vi "Teleop.vi"(10 "Match Info":T1={"Autonomous Elapsed Seconds"=0.0, "TeleOp Elapsed Seconds"=0.0, "Disabled Elapsed Seconds"=0.0, "Visited Autonomous"=FALSE, "Visited TeleOp"=FALSE, "Visited Disabled"=FALSE, "Autonomous Settings"={"Autonomous Style"=enum."Independent", "VI Refnum"=refnum}}, 11 "Call Context":T2) -> ()   [LabVIEW 2019]
doc: "This VI is called for each TeleOp packet received from the DS where the robot is not disabled. It is often used to read from the joysticks and update I/O or to update setpoints for timed control loops. It should complete and return within 20 milliseconds or it may miss DS packets."
uses:
  ArgosLib/ArgosLib.lvlib
  InfiniteRechargeSrc/Global_Var-RefNum/JoystickControls.vi
  InfiniteRechargeSrc/TypeDefs/JoystickControl.ctl
  <vilib>/Rock Robotics/WPI/DriverStation/WPI_DriverStationMatch Info.ctl
  <vilib>/Rock Robotics/WPI/DriverStation/WPI_DriverStationDerivedRobotMode.ctl
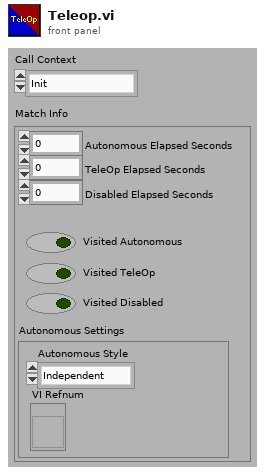
[diagram p1: front panel]
types:
  T1 = typedef "WPI_DriverStationMatch Info.ctl" = cluster{"Autonomous Elapsed Seconds":dbl, "TeleOp Elapsed Seconds":dbl, "Disabled Elapsed Seconds":dbl, "Visited Autonomous":bool, "Visited TeleOp":bool, "Visited Disabled":bool, "Autonomous Settings":cluster{"Autonomous Style":enum16{"Iterative", "Independent"}, "VI Refnum":refnum<vi>}}
  T2 = typedef "WPI_DriverStationDerivedRobotMode.ctl" = enum16{"Init", "Execute", "Stop"}
  T3 = typedef "JoystickControl.ctl" = cluster{"A":bool, "B":bool, "X":bool, "Y":bool, "LB":bool, "RB":bool, "LJ":bool, "RJ":bool, "Back":bool, "Start":bool, "Top":bool, "Right":bool, "Bottom":bool, "Left":bool, "LT":dbl, "RT":dbl, "LX":dbl, "LY":dbl, "RX":dbl, "RY":dbl, "A 2":bool, "B 2":bool, "X 2":bool, "Y 2":bool, "LB 2":bool, "RB 2":bool, "LJ 2":bool, "RJ 2":bool, "Back 2":bool, "Start 2":bool, "Top 2":bool, "Right 2":bool, "Bottom 2":bool, "Left 2":bool, "LT 2":dbl, "RT 2":dbl, "LX 2":dbl, "LY 2":dbl, "RX 2":dbl, "RY 2":dbl}
  T4 = typedef "JoystickRefNums.ctl" = cluster{"Joystick0":T5, "Joystick1":T5}
  T5 = typedef "WPI_JoystickDevRef.ctl" = cluster{"Device":T6}
  T6 = typedef "WPI_JoystickDeviceEnum.ctl" = enum16{"USB 0", "USB 1", "USB 2", "USB 3", "USB 4", "USB 5"}
  T7 = typedef "ArgosLib.lvlib/XBoxAxes_Type.ctl" = cluster{"Left_Trigger":dbl, "Right_Trigger ":dbl, "Left_X":dbl, "Left_Y":dbl, "Right_X":dbl, "Right_Y":dbl}
  T8 = typedef "ArgosLib.lvlib/XBoxButtons_Type.ctl" = cluster{"A":bool, "B":bool, "X":bool, " Y":bool, "LB":bool, " RB":bool, "Left_Thumb_Button":bool, "Right_Thumb_Button":bool, "Back":bool, "Start":bool, "Top":bool, "Right":bool, "Bottom":bool, "Left":bool}
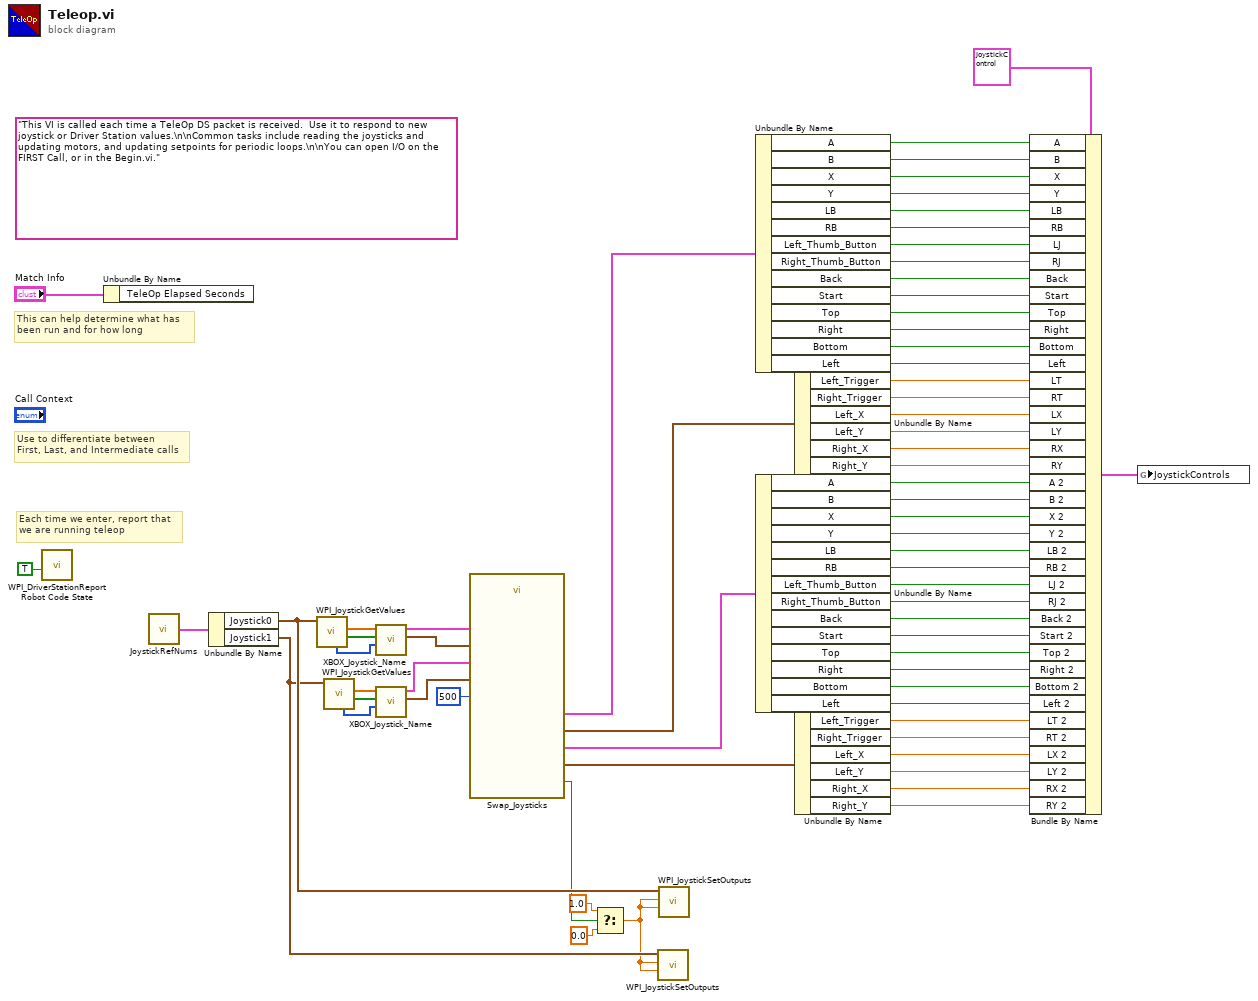
[diagram p0: block diagram]
diagram:
  (unwired) "This VI is called each time a TeleOp DS packet is received.  Use it to respond to new joystick or Driver Station values.\n\nCommon tasks include reading the joysticks and updating motors, and updating setpoints for periodic loops.\n\nYou can open I/O on the FIRST Call, or in the Begin.vi."
  # "Each time we enter, report that\nwe are running teleop"
  # "Use to differentiate between\nFirst, Last, and Intermediate calls"
  # "This can help determine what has\nbeen run and for how long"
  n1 = call <vilib>:"WPI_DriverStationReport Robot Code State.vi"("TeleOp"=TRUE ("Autonomous")) -> ()  [unwired: 10 in, 1 out]
  n2 = Unbundle By Name("Match Info") -> ()  [unwired: 1 out]
  n3 = call "JoystickRefNums.vi"() -> ("JoystickRefNums"=w64:T4)  [unwired: 1 in]
  n4 = Unbundle By Name(w64) -> ("Joystick0"=w53:T5, "Joystick1"=w52:T5)
  n5 = call <vilib>:"WPI_JoystickGetValues.vi"("JoystickDevRef"=w53) -> ("Buttons"=w59:bool[], "Axes"=w60:dbl[], "POVs"=w58:i16[])  [unwired: 6 in, 2 out]
  n6 = call <vilib>:"WPI_JoystickGetValues.vi"("JoystickDevRef"=w52) -> ("Buttons"=w62:bool[], "Axes"=w63:dbl[], "POVs"=w61:i16[])  [unwired: 6 in, 2 out]
  n7 = call "XBOX_Joystick_Name.vi"("POVs"=w58, "Buttons"=w59, "Axes"=w60) -> ("Named Axes"=w56:T7, "Named Buttons"=w57:T8)  [unwired: 7 in]
  n8 = call "XBOX_Joystick_Name.vi"("POVs"=w61, "Buttons"=w62, "Axes"=w63) -> ("Named Axes"=w54:T7, "Named Buttons"=w55:T8)  [unwired: 7 in]
  n9 = call "Swap_Joysticks.vi"("Hold Time(ms)"=u32 500, "Axes 1 In"=w54, "Buttons 1"=w55, "Axes 0 in"=w56, "Buttons 0"=w57) -> ("Axes 1 out"=w44:T7, "Buttons 1 out"=w45:T8, "Axes 0 out"=w46:T7, "Buttons 0 Out"=w47:T8, "Swap?"=w51:bool)
  n10 = Select(t=sgl 1.0, s=w51, f=sgl 0.0) -> (s? t:f=w48:sgl)
  n11 = call <vilib>:"WPI_JoystickSetOutputs.vi"("Right Rumble"=w48, "Left Rumble"=w48, "JoystickDevRef"=w52) -> ()  [unwired: 7 in, 2 out]
  n12 = call <vilib>:"WPI_JoystickSetOutputs.vi"("Right Rumble"=w48, "Left Rumble"=w48, "JoystickDevRef"=w53) -> ()  [unwired: 7 in, 2 out]
  n13 = Unbundle By Name(w47) -> ("A"=w41:bool, "B"=w40:bool, "X"=w39:bool, "Y"=w38:bool, "LB"=w37:bool, "RB"=w36:bool, "Left_Thumb_Button"=w35:bool, "Right_Thumb_Button"=w34:bool, "Back"=w33:bool, "Start"=w32:bool, "Top"=w31:bool, "Right"=w30:bool, "Bottom"=w29:bool, "Left"=w28:bool)
  n14 = Unbundle By Name(w45) -> ("A"=w21:bool, "B"=w20:bool, "X"=w19:bool, "Y"=w18:bool, "LB"=w17:bool, "RB"=w16:bool, "Left_Thumb_Button"=w15:bool, "Right_Thumb_Button"=w14:bool, "Back"=w13:bool, "Start"=w12:bool, "Top"=w11:bool, "Right"=w10:bool, "Bottom"=w9:bool, "Left"=w8:bool)
  n15 = Unbundle By Name(w46) -> ("Left_Trigger"=w27:dbl, "Right_Trigger"=w26:dbl, "Left_X"=w25:dbl, "Left_Y"=w24:dbl, "Right_X"=w23:dbl, "Right_Y"=w22:dbl)
  n16 = Unbundle By Name(w44) -> ("Left_Trigger"=w7:dbl, "Right_Trigger"=w6:dbl, "Left_X"=w5:dbl, "Left_Y"=w4:dbl, "Right_X"=w3:dbl, "Right_Y"=w2:dbl)
  n17 = Bundle By Name(cluster=T3 {"A"=FALSE, "B"=FALSE, "X"=FALSE, "Y"=FALSE, "LB"=FALSE, "RB"=FALSE, "LJ"=FALSE, "RJ"=FALSE, "Back"=FALSE, "Start"=FALSE, "Top"=FALSE, "Right"=FALSE, "Bottom"=FALSE, "Left"=FALSE, "LT"=0.0, "RT"=0.0, "LX"=0.0, "LY"=0.0, "RX"=0.0, "RY"=0.0, "A 2"=FALSE, "B 2"=FALSE, "X 2"=FALSE, "Y 2"=FALSE, "LB 2"=FALSE, "RB 2"=FALSE, "LJ 2"=FALSE, "RJ 2"=FALSE, "Back 2"=FALSE, "Start 2"=FALSE, "Top 2"=FALSE, "Right 2"=FALSE, "Bottom 2"=FALSE, "Left 2"=FALSE, "LT 2"=0.0, "RT 2"=0.0, "LX 2"=0.0, "LY 2"=0.0, "RX 2"=0.0, "RY 2"=0.0} ("JoystickControls"), "A"=w41, "B"=w40, "X"=w39, "Y"=w38, "LB"=w37, "RB"=w36, "LJ"=w35, "RJ"=w34, "Back"=w33, "Start"=w32, "Top"=w31, "Right"=w30, "Bottom"=w29, "Left"=w28, "LT"=w27, "RT"=w26, "LX"=w25, "LY"=w24, "RX"=w23, "RY"=w22, "A 2"=w21, "B 2"=w20, "X 2"=w19, "Y 2"=w18, "LB 2"=w17, "RB 2"=w16, "LJ 2"=w15, "RJ 2"=w14, "Back 2"=w13, "Start 2"=w12, "Top 2"=w11, "Right 2"=w10, "Bottom 2"=w9, "Left 2"=w8, "LT 2"=w7, "RT 2"=w6, "LX 2"=w5, "LY 2"=w4, "RX 2"=w3, "RY 2"=w2) -> (w1:T3)
  n18 = global write "JoystickControls.vi" "JoystickControls"(w1) -> ()
